vi "Anlagengrenzwerte pruefen - cRIO.vi"(6 "Aktion":T1, 9 "Wert":sgl, 10 "Anlagen-Parametername":T2) -> (0 "AbschMax":bool, 1 "AbschMin":bool, 2 "WarnMax":bool, 3 "WarnMin":bool, 5 "F.Br.":bool)   [LabVIEW 2020, in "Stoermeldungen.lvlib"]
uses:
  Stoermeldungen.lvlib
  Seiten/Anlagengrenzwerte/Anlagen-Parameternamen.ctl
  Aktion Anlagengrenzen pruefen.ctl
  Konfig-Dateien/FGV Betriebsdaten Aktionen.ctl
  Aktion Heizung Uebertemperatur.ctl
  Allgemein/FGV Zustaende Aktionen.ctl
  Funktionstasten/Zustaende.ctl
  Verwaltung/FGV IN Aktionen.ctl
  Allgemein/Allgemein.lvlib
  Funktionstasten/Funktionstasten.lvlib
  Konfig-Dateien/Konfig-Dateien.lvlib
  Verwaltung/Verwaltung - cRIO.lvlib
  Seiten/Anlagengrenzwerte/Anlagengrenzwerte.lvlib
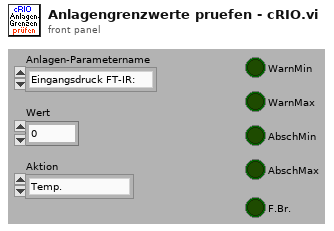
[diagram p1: front panel]
types:
  T1 = typedef "Stoermeldungen.lvlib/Aktion Anlagengrenzen pruefen.ctl" = enum16{"Temp.", "HKL", "Druck", "SS Temp."}
  T2 = typedef "Anlagengrenzwerte.lvlib/Anlagen-Parameternamen.ctl" = enum16{"Eingangsdruck FT-IR:", "Durchfluss FT-IR:", "Durchfluss CalGas", "Druck Ausgang", "Druck Kalter Block", "Heizleitung intern", "Heizleitung zu FT-IR", "Heizung Filter:", "Heizung Pumpe:", "HL Extern SP1", "HL Extern SP2", "FT-IR Messzelle", "Schaltschrank", "Gaskühler"}
  T3 = typedef "Konfig-Dateien.lvlib/FGV Betriebsdaten Aktionen.ctl" = enum16{"lesen", "Anlagengrenzw.", "PID Param.", "Sonstige", "Sensor Para."}
  T4 = typedef "Anlagengrenzwerte.lvlib/Anlagen-Grenzwerte Anzeige.ctl" = cluster{"Eingangsdruck FT-IR:":T5, "Durchfluss FT-IR:":T5, "Durchfluss CalGas:":T5, "Druck Ausgang:":T5, "Druck Kalter Block:":T5, "Heizleitungen intern:":T5, "Heizleitung zu FT-IR:":T5, "Heizung Filterblock:":T5, "Heizung Pumpe:":T5, "Heizleitung Extern SP1:":T5, "Heizleitung Extern SP2:":T5, "FT-IR Heizung Messzelle:":T5, "Schaltschranktemperatur:":T5, "Gaskühler:":T5}
  T5 = typedef "Anlagengrenzwerte.lvlib/Anlagen-Parameter Anzeige.ctl" = cluster{"Sollwert":sgl, "Warn-Min":sgl, "Warn-Max":sgl, "Abschalt-Min":sgl, "Abschalt-Max":sgl, "Regler":u16}
  T6 = typedef "Stoermeldungen.lvlib/Aktion Heizung Uebertemperatur.ctl" = enum16{"lesen", "prüfen", "rücksetzen"}
  T7 = typedef "Funktionstasten.lvlib/Zustaende.ctl" = enum16{"Standby", "Pause", "Eco", "Messen", "Kalibrieren", "Spülen Filter", "Spülen Leitung", "Umgebungsluft", "0-Gas", "Cal-Gas", "CG zu PNS", "-------------", "Init 1", "Init 2", "Init 3", "Init 4", "Messen vorbereiten", "Messen durchführen", "Exit"}
  T8 = typedef "Allgemein.lvlib/FGV Zustaende Aktionen.ctl" = enum16{"lesen", "Zustand PC", "Zustand cRIO", "Bildnummer", "Samplepoint", "Sysloglevel"}
  T9 = typedef "Verwaltung - cRIO.lvlib/FGV IN Aktionen.ctl" = enum16{"lesen", "DI", "AI", "Fühler Br.", "TC", "Fühler Br. TC"}
  T10 = typedef "Verwaltung - cRIO.lvlib/Fuehler Bruch AI.ctl" = cluster{"AI0: Durchfluss FT-IR":bool, "AI1: Druck Ausgang":bool, "AI2: Umgebungsdruck":bool, "AI3: Druck FT-IR":bool, "AI4: Druck CalGas":bool, "AI5: Reserve":bool, "AI6: Reserve":bool, "AI7: Reserve":bool}
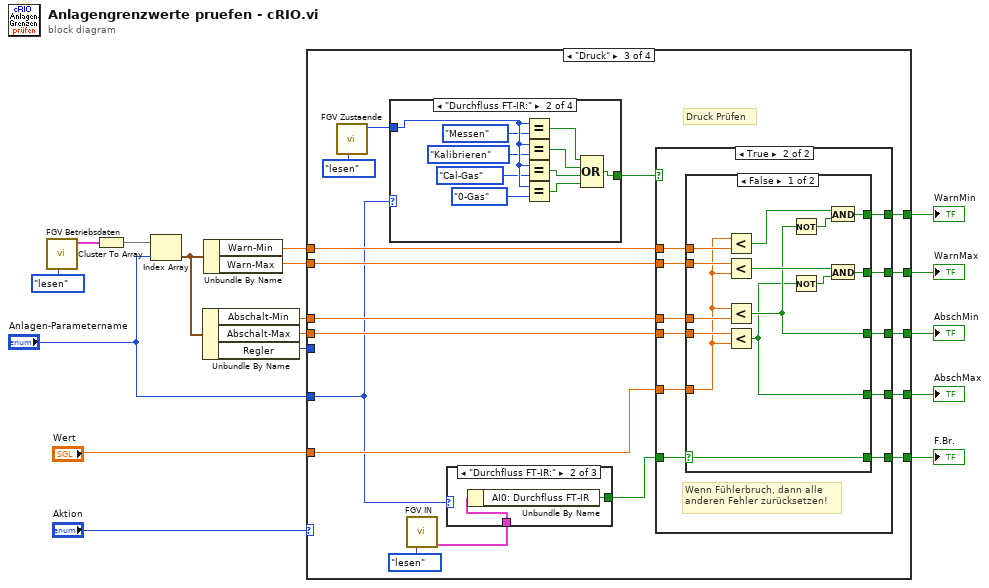
[diagram p0: block diagram]
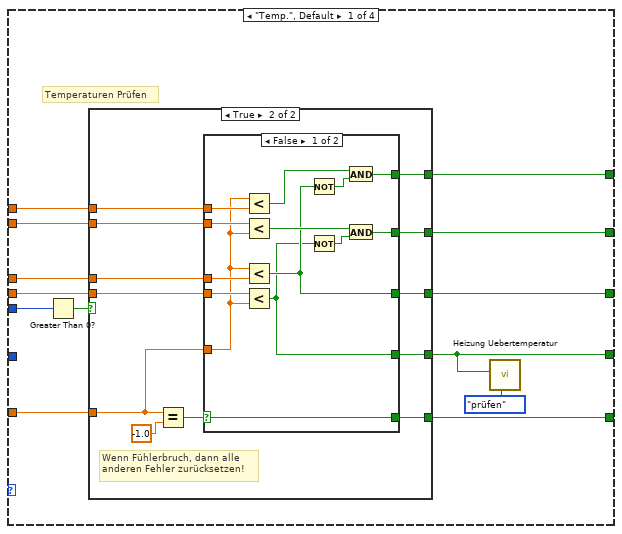
[diagram p2: hidden frame]
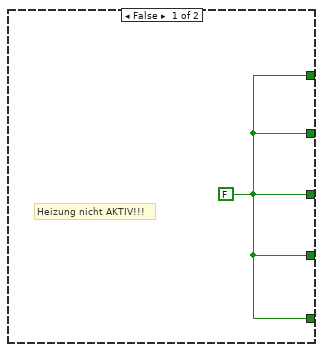
[diagram p3: hidden frame]
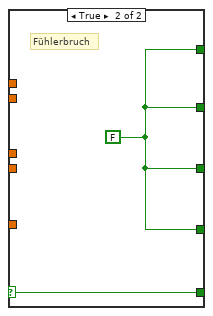
[diagram p4: hidden frame]
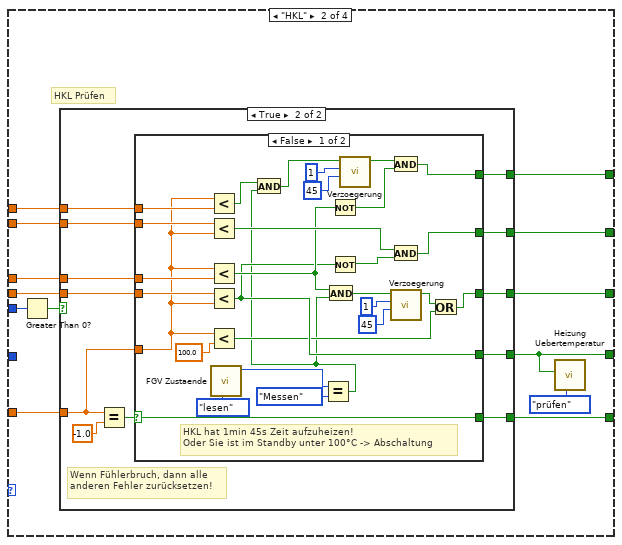
[diagram p5: hidden frame]
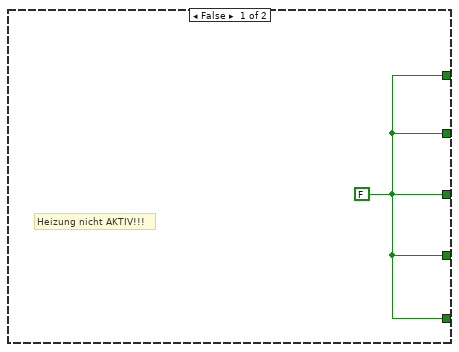
[diagram p6: hidden frame]
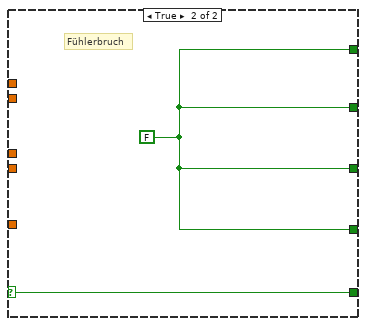
[diagram p7: hidden frame]
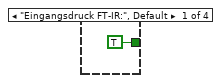
[diagram p8: hidden frame]
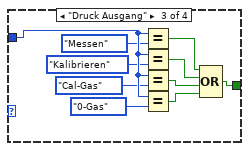
[diagram p9: hidden frame]
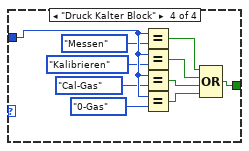
[diagram p10: hidden frame]
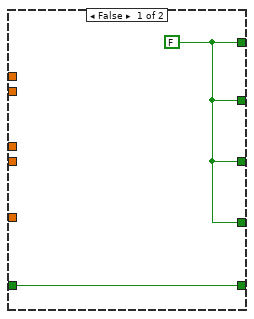
[diagram p11: hidden frame]
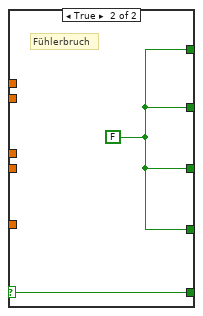
[diagram p12: hidden frame]
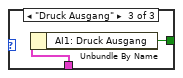
[diagram p14: hidden frame]
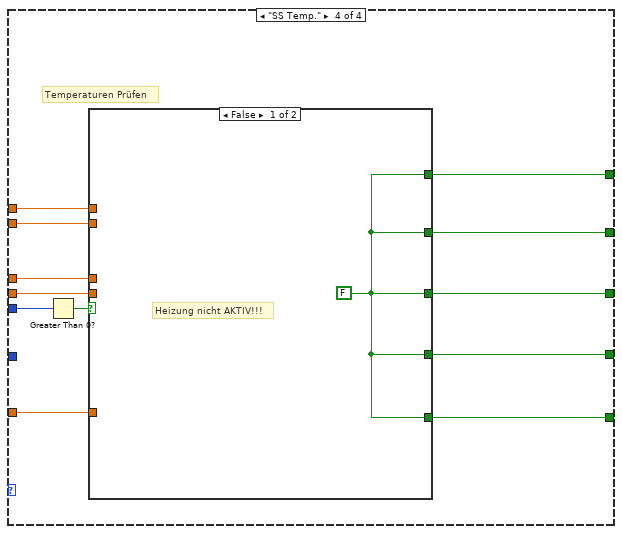
[diagram p15: hidden frame]
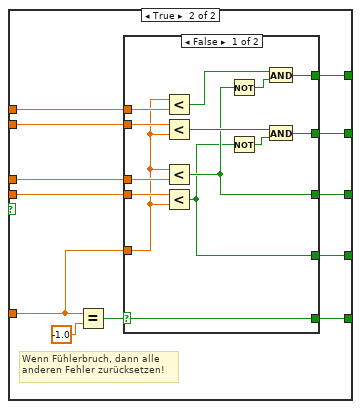
[diagram p16: hidden frame]
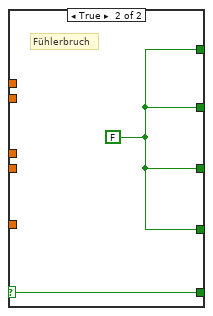
[diagram p17: hidden frame]
diagram:
  n1 = call "FGV Betriebsdaten.vi"("Aktionen"=FGV_Betriebsdaten_Aktionen."lesen") -> ("Anlagen-Grenzwerte"=w1:T4)  [unwired: 7 in, 3 out]
  n2 = Cluster To Array(cluster=w1) -> (array=w17:T5[])
  n3 = Index Array(array=w17, index="Anlagen-Parametername") -> (element=w16:T5)
  n4 = Unbundle By Name(w16) -> ("Abschalt-Min"=w13:sgl, "Abschalt-Max"=w12:sgl, "Regler"=w4:u16)
  n5 = Unbundle By Name(w16) -> ("Warn-Min"=w15:sgl, "Warn-Max"=w14:sgl)
  n6 = case shown="\"Druck\"" "Aktion" {
    tunnel: w15 -> [w30 w72 w127 w209]
    tunnel: w14 -> [w29 w71 w126 w208]
    tunnel: w13 -> [w28 w70 w125 w207]
    tunnel: w12 -> [w27 w69 w124 w206]
    tunnel: "Wert" -> [w26 w68 w123 w205]
    tunnel: [w25 w67 w132 w204] -> w9
    tunnel: [w24 w66 w131 w203] -> w8
    tunnel: [w23 w65 w130 w202] -> w7
    tunnel: [w20 w63 w129 w200] -> w6
    tunnel: [w22 w64 w128 w201] -> w5
    tunnel: w4 -> [w19 w61 _ w199]
    tunnel: "Anlagen-Parametername" -> [_ _ w122 _]
    frame "Temp.", Default {
      # "Temperaturen Prüfen"
      n7 = Greater Than 0?(x=w19) -> (x > 0?=w18:bool)
      n8 = case shown="True" w18 {
        tunnel: w30 -> [_ w43]
        tunnel: w29 -> [_ w42]
        tunnel: w28 -> [_ w41]
        tunnel: w27 -> [_ w40]
        tunnel: w26 -> [_ w37]
        tunnel: [w31 w36] -> w25
        tunnel: [w31 w35] -> w24
        tunnel: [w31 w34] -> w23
        tunnel: [w31 w33] -> w22
        tunnel: [w31 w32] -> w20
        frame False {
          w31 = FALSE
          # "Heizung nicht AKTIV!!!"
        }
        frame True {
          # "Wenn Fühlerbruch, dann alle \nanderen Fehler zurücksetzen!"
          n9 = Equal?(x=w37, y=sgl -1.0) -> (x = y?=w38:bool)
          n10 = case shown="False" w38 {
            selector: w38 -> [w44 w59]
            tunnel: w43 -> [w57 _]
            tunnel: w42 -> [w56 _]
            tunnel: w41 -> [w55 _]
            tunnel: w40 -> [w54 _]
            tunnel: [w49 w58] -> w36
            tunnel: [w48 w58] -> w35
            tunnel: [w47 w58] -> w34
            tunnel: [w46 w58] -> w32
            tunnel: w37 -> [w45 _]
            tunnel: [w44 w59] -> w33
            frame False {
              n11 = Less?(x=w45, y=w57) -> (x < y?=w53:bool)
              n12 = Less?(x=w56, y=w45) -> (x < y?=w50:bool)
              n13 = Less?(x=w45, y=w55) -> (x < y?=w47:bool)
              n14 = Less?(x=w54, y=w45) -> (x < y?=w46:bool)
              n15 = Not(x=w47) -> (.not. x?=w52:bool)
              n16 = Not(x=w46) -> (.not. x?=w51:bool)
              n17 = And(x=w53, y=w52) -> (x .and. y?=w49:bool)
              n18 = And(x=w50, y=w51) -> (x .and. y?=w48:bool)
            }
            frame True {
              w58 = FALSE
              # "Fühlerbruch"
            }
          }
        }
      }
      n19 = call "Heizung Uebertemperatur.vi"("Aktionen"=Aktion_Heizung_Uebertemperatur."prüfen", "Heizung Übertemperatur"=w20) -> ()  [unwired: 8 in, 2 out]
    }
    frame "HKL" {
      # "HKL Prüfen"
      n20 = Greater Than 0?(x=w61) -> (x > 0?=w60:bool)
      n21 = case shown="True" w60 {
        tunnel: w72 -> [_ w83]
        tunnel: w71 -> [_ w82]
        tunnel: w70 -> [_ w81]
        tunnel: w69 -> [_ w80]
        tunnel: w68 -> [_ w79]
        tunnel: [w73 w78] -> w67
        tunnel: [w73 w77] -> w66
        tunnel: [w73 w76] -> w65
        tunnel: [w73 w75] -> w64
        tunnel: [w73 w74] -> w63
        frame False {
          w73 = FALSE
          # "Heizung nicht AKTIV!!!"
        }
        frame True {
          # "Wenn Fühlerbruch, dann alle \nanderen Fehler zurücksetzen!"
          n22 = Equal?(x=w79, y=sgl -1.0) -> (x = y?=w84:bool)
          n23 = case shown="False" w84 {
            selector: w84 -> [w105 w116]
            tunnel: w83 -> [w114 _]
            tunnel: w82 -> [w113 _]
            tunnel: w81 -> [w112 _]
            tunnel: w80 -> [w111 _]
            tunnel: [w107 w115] -> w78
            tunnel: [w106 w115] -> w77
            tunnel: [w91 w115] -> w76
            tunnel: [w95 w115] -> w74
            tunnel: w79 -> [w94 _]
            tunnel: [w105 w116] -> w75
            frame False {
              # "HKL hat 1min 45s Zeit aufzuheizen!\nOder Sie ist im Standby unter 100°C -> Abschaltung"
              n24 = Less?(x=w94, y=w114) -> (x < y?=w101:bool)
              n25 = Less?(x=w113, y=w94) -> (x < y?=w108:bool)
              n26 = Less?(x=w94, y=w112) -> (x < y?=w103:bool)
              n27 = Less?(x=w111, y=w94) -> (x < y?=w95:bool)
              n28 = Less?(x=w94, y=sgl 100.0) -> (x < y?=w90:bool)
              n29 = call "FGV Zustaende.vi"("Aktionen"=FGV_Zustaende_Aktionen."lesen") -> ("Zustand PC"=w87:T7)  [unwired: 6 in, 4 out]
              n30 = Equal?(x=w87, y=Zustaende."Messen") -> (x = y?=w89:bool)
              n31 = And(x=w101, y=w89) -> (x .and. y?=w100:bool)
              n32 = And(x=w103, y=w89) -> (x .and. y?=w102:bool)
              n33 = Not(x=w103) -> (.not. x?=w110:bool)
              n34 = Not(x=w95) -> (.not. x?=w109:bool)
              n35 = call "Verzoegerung.vi"("sec"=u16 45, "min"=u16 1, "Startsignal"=w100) -> ("Zeit abgelaufen?"=w104:bool)  [unwired: 7 in, 1 out]
              n36 = And(x=w104, y=w110) -> (x .and. y?=w107:bool)
              n37 = And(x=w108, y=w109) -> (x .and. y?=w106:bool)
              n38 = call "Verzoegerung.vi"("sec"=u16 45, "min"=u16 1, "Startsignal"=w102) -> ("Zeit abgelaufen?"=w92:bool)  [unwired: 7 in, 1 out]
              n39 = Or(x=w92, y=w90) -> (x .or. y?=w91:bool)
            }
            frame True {
              w115 = FALSE
              # "Fühlerbruch"
            }
          }
        }
      }
      n40 = call "Heizung Uebertemperatur.vi"("Aktionen"=Aktion_Heizung_Uebertemperatur."prüfen", "Heizung Übertemperatur"=w63) -> ()  [unwired: 8 in, 2 out]
    }
    frame "Druck" {
      # "Druck Prüfen"
      n41 = call "FGV Zustaende.vi"("Aktionen"=FGV_Zustaende_Aktionen."lesen") -> ("Zustand PC"=w117:T7)  [unwired: 6 in, 4 out]
      n42 = case shown="\"Durchfluss FT-IR:\"" w122 {
        tunnel: w117 -> [_ w139 w149 w159]
        tunnel: [TRUE w144 w154 w164] -> w121
        frame "Eingangsdruck FT-IR:", Default {
        }
        frame "Durchfluss FT-IR:" {
          n43 = Equal?(x=w139, y=Zustaende."Messen" ("Zustand PC")) -> (x = y?=w143:bool)
          n44 = Equal?(x=w139, y=Zustaende."Kalibrieren" ("Zustand PC")) -> (x = y?=w142:bool)
          n45 = Equal?(x=w139, y=Zustaende."Cal-Gas" ("Zustand PC")) -> (x = y?=w141:bool)
          n46 = Equal?(x=w139, y=Zustaende."0-Gas" ("Zustand PC")) -> (x = y?=w140:bool)
          n47 = Compound Arithmetic op=OR(w143, w142, w141, w140) -> (w144:bool)
        }
        frame "Druck Ausgang" {
          n48 = Equal?(x=w149, y=Zustaende."Messen" ("Zustand PC")) -> (x = y?=w153:bool)
          n49 = Equal?(x=w149, y=Zustaende."Kalibrieren" ("Zustand PC")) -> (x = y?=w152:bool)
          n50 = Equal?(x=w149, y=Zustaende."Cal-Gas" ("Zustand PC")) -> (x = y?=w151:bool)
          n51 = Equal?(x=w149, y=Zustaende."0-Gas" ("Zustand PC")) -> (x = y?=w150:bool)
          n52 = Compound Arithmetic op=OR(w153, w152, w151, w150) -> (w154:bool)
        }
        frame "Druck Kalter Block" {
          n53 = Equal?(x=w159, y=Zustaende."Messen" ("Zustand PC")) -> (x = y?=w163:bool)
          n54 = Equal?(x=w159, y=Zustaende."Kalibrieren" ("Zustand PC")) -> (x = y?=w162:bool)
          n55 = Equal?(x=w159, y=Zustaende."Cal-Gas" ("Zustand PC")) -> (x = y?=w161:bool)
          n56 = Equal?(x=w159, y=Zustaende."0-Gas" ("Zustand PC")) -> (x = y?=w160:bool)
          n57 = Compound Arithmetic op=OR(w163, w162, w161, w160) -> (w164:bool)
        }
      }
      n58 = call "FGV IN.vi"("Aktion"=FGV_IN_Aktionen."lesen") -> ("Fühler Bruch AI"=w118:T10)  [unwired: 10 in, 4 out]
      n59 = case shown="\"Durchfluss FT-IR:\"" w122 {
        tunnel: w118 -> [_ w195 w197]
        tunnel: [_ w194 w196] -> w133
        frame "Eingangsdruck FT-IR:", Default {
        }
        frame "Durchfluss FT-IR:" {
          n60 = Unbundle By Name(w195) -> ("AI0: Durchfluss FT-IR"=w194:bool)
        }
        frame "Druck Ausgang" {
          n61 = Unbundle By Name(w197) -> ("AI1: Druck Ausgang"=w196:bool)
        }
      }
      n62 = case shown="True" w121 {
        tunnel: w133 -> [w165 w177]
        tunnel: [w166 w176] -> w132
        tunnel: [w166 w175] -> w131
        tunnel: [w166 w174] -> w130
        tunnel: [w166 w173] -> w129
        tunnel: [w165 w172] -> w128
        tunnel: w127 -> [_ w171]
        tunnel: w126 -> [_ w170]
        tunnel: w125 -> [_ w169]
        tunnel: w124 -> [_ w168]
        tunnel: w123 -> [_ w167]
        frame False {
          w166 = FALSE
        }
        frame True {
          # "Wenn Fühlerbruch, dann alle \nanderen Fehler zurücksetzen!"
          n63 = case shown="False" w177 {
            selector: w177 -> [w178 w193]
            tunnel: w171 -> [w191 _]
            tunnel: w170 -> [w190 _]
            tunnel: w169 -> [w189 _]
            tunnel: w168 -> [w188 _]
            tunnel: [w183 w192] -> w176
            tunnel: [w182 w192] -> w175
            tunnel: [w181 w192] -> w174
            tunnel: [w180 w192] -> w173
            tunnel: w167 -> [w179 _]
            tunnel: [w178 w193] -> w172
            frame False {
              n64 = Less?(x=w179, y=w191) -> (x < y?=w187:bool)
              n65 = Less?(x=w190, y=w179) -> (x < y?=w184:bool)
              n66 = Less?(x=w179, y=w189) -> (x < y?=w181:bool)
              n67 = Less?(x=w188, y=w179) -> (x < y?=w180:bool)
              n68 = Not(x=w181) -> (.not. x?=w186:bool)
              n69 = Not(x=w180) -> (.not. x?=w185:bool)
              n70 = And(x=w187, y=w186) -> (x .and. y?=w183:bool)
              n71 = And(x=w184, y=w185) -> (x .and. y?=w182:bool)
            }
            frame True {
              w192 = FALSE
              # "Fühlerbruch"
            }
          }
        }
      }
    }
    frame "SS Temp." {
      # "Temperaturen Prüfen"
      n72 = Greater Than 0?(x=w199) -> (x > 0?=w198:bool)
      n73 = case shown="False" w198 {
        tunnel: w209 -> [_ w222]
        tunnel: w208 -> [_ w221]
        tunnel: w207 -> [_ w220]
        tunnel: w206 -> [_ w219]
        tunnel: w205 -> [_ w216]
        tunnel: [w210 w215] -> w204
        tunnel: [w210 w214] -> w203
        tunnel: [w210 w213] -> w202
        tunnel: [w210 w212] -> w201
        tunnel: [w210 w211] -> w200
        frame False {
          w210 = FALSE
          # "Heizung nicht AKTIV!!!"
        }
        frame True {
          # "Wenn Fühlerbruch, dann alle \nanderen Fehler zurücksetzen!"
          n74 = Equal?(x=w216, y=sgl -1.0) -> (x = y?=w217:bool)
          n75 = case shown="False" w217 {
            selector: w217 -> [w223 w238]
            tunnel: w222 -> [w236 _]
            tunnel: w221 -> [w235 _]
            tunnel: w220 -> [w234 _]
            tunnel: w219 -> [w233 _]
            tunnel: [w228 w237] -> w215
            tunnel: [w227 w237] -> w214
            tunnel: [w226 w237] -> w213
            tunnel: [w225 w237] -> w211
            tunnel: w216 -> [w224 _]
            tunnel: [w223 w238] -> w212
            frame False {
              n76 = Less?(x=w224, y=w236) -> (x < y?=w232:bool)
              n77 = Less?(x=w235, y=w224) -> (x < y?=w229:bool)
              n78 = Less?(x=w224, y=w234) -> (x < y?=w226:bool)
              n79 = Less?(x=w233, y=w224) -> (x < y?=w225:bool)
              n80 = Not(x=w226) -> (.not. x?=w231:bool)
              n81 = Not(x=w225) -> (.not. x?=w230:bool)
              n82 = And(x=w232, y=w231) -> (x .and. y?=w228:bool)
              n83 = And(x=w229, y=w230) -> (x .and. y?=w227:bool)
            }
            frame True {
              w237 = FALSE
              # "Fühlerbruch"
            }
          }
        }
      }
    }
  }
  "WarnMin" <- w9
  "WarnMax" <- w8
  "AbschMin" <- w7
  "AbschMax" <- w6
  "F.Br." <- w5
